vi "Get Timer Status.vi"(8 "error in (no error)":errorcluster, 11 "timer":T1) -> (0 "error out":errorcluster, 1 "Total time (s)":dbl format="%.3f", 2 "# waiting":i32, 3 "timer out":T1, 4 "Running":bool, 5 "name out":string)   [LabVIEW 2011]
doc: "Returns current status information of the timer.\n\n© Copyright 1999\nCal-Bay Systems, Inc.\nwritten by James Kring"
uses:
  Timer Refnum.ctl
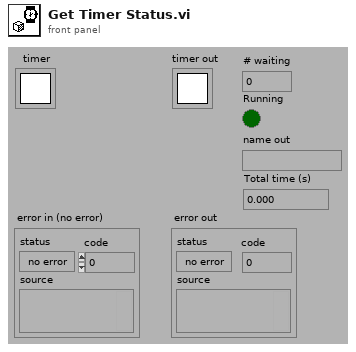
[diagram p1: front panel]
types:
  T1 = typedef "Timer Refnum.ctl" = refnum<k1>
  T2 = enum16{"open ref", "lookup ref", "close ref", "test ref", "start", "stop", "wait", "reset", "increment # waiting", "decrement #waiting"}
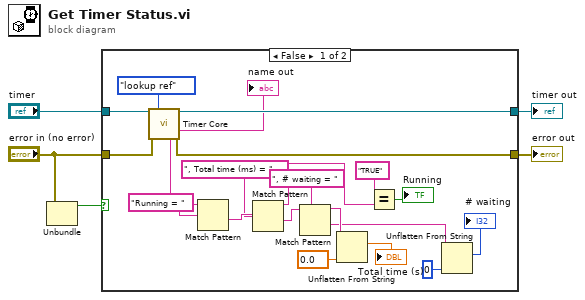
[diagram p0: block diagram]
diagram:
  n1 = Unbundle("error in (no error)") -> ("status"=w4:bool)  [unwired: 2 out]
  n2 = case shown="False" w4 {
    tunnel: "timer" -> [w26 w27]
    tunnel: [w25 w27] -> w1
    tunnel: "error in (no error)" -> [w23 w28]
    tunnel: [w24 w28] -> w2
    frame False {
      n3 = call "Timer Core.vi"("timer"=w26, "function"=T2."lookup ref", "error in (no error)"=w23) -> ("timer out"=w25:T1, "name out"=→"name out":string, "message out"=w20:string, "error out"=w24:errorcluster)  [unwired: 6 in, 3 out]
      n4 = Match Pattern(string=w20, regular expression="Running = " ("Format String")) -> (after substring=w18:string)  [unwired: 1 in, 3 out]
      n5 = Match Pattern(string=w18, regular expression=", Total time (ms) = " ("Format String")) -> (before substring=w10:string, after substring=w12:string)  [unwired: 1 in, 2 out]
      n6 = Match Pattern(string=w12, regular expression=", # waiting = ") -> (before substring=w8:string, after substring=w7:string)  [unwired: 1 in, 2 out]
      n7 = Unflatten From String(type=0.0 ("Total time (ms)"), binary string=w8) -> (value=→"Total time (s)":dbl)  [unwired: 3 in, 2 out]
      n8 = Equal?(x="TRUE", y=w10) -> (x = y?=→"Running":bool)
      n9 = Unflatten From String(type=0 ("Total time (ms)"), binary string=w7) -> (value=→"# waiting":i32)  [unwired: 3 in, 2 out]
    }
    frame True {
    }
  }
  "timer out" <- w1
  "error out" <- w2
